vi "Spectral Integration Threshold Ranging.vi"() -> ()   [LabVIEW 2018]
uses:
  <instrlib>/Ocean Optics 2000 4000/Ocean Optics 2000 4000.lvlib
panel:
  out "error out":errorcluster
  in  "Threshold":dbl format="%#_13g"
  out "Peak Wavelength vs Time":cluster{"X":dbl[], "Y":dbl[]}[](graph) caption="XY Graph"
  out "Experiment Length":enum32{"Short", "Long"}(tab)=enum."Long"
  in  "Runtime, s":dbl=20.0
  in  "Maximum Measurement Rate, ms":u32
  in  "Runtime, mins":dbl=20.0
  in  "Maximum Measurement Rate, s":u32=30
  in  "Experiment Length":bool=TRUE
  out "Peak Wavelength Change":cluster{dbl[], dbl[]}(graph)
  out "Integration Change":cluster{dbl[], dbl[]}(graph)
  out "Fitted Target Waveform":cluster{dbl[], dbl[]}(graph)
  out "Target Waveform":cluster{dbl[], dbl[]}(graph)
  in  "?":bool
  out "End Index":i32
  out "Length":i32
  out "Start Index":i32
  out "Calculated Dlambda":dbl[][](array[numeric])
  out "Current Measurement Index":i32
  in  "Wavelength Range":bool
  out "Number of Measurements":dbl
  out "Integration Time":u32
  in  "Intensity Averaging":bool
  out "Integration vs Time":cluster{"Y":dbl[], "Y":dbl[]}[](graph)
  out "Log Data":dbl[][](array[numeric])
  in  "Data Log":bool caption="Log Data"
  in  "File Name":string="Example.xls" caption="add .xls for excel or .tdms, etc"
  in  "Number of Spectrum (Max 5)":i32=5
  in  "Integration Time, ms":dbl=100.0
  in  "Enable Strobe":bool
  out "Spectral Waveform":cluster{dbl[], dbl[]}(graph)
  in  "VISA resource name":refnum<visa-resource-name>
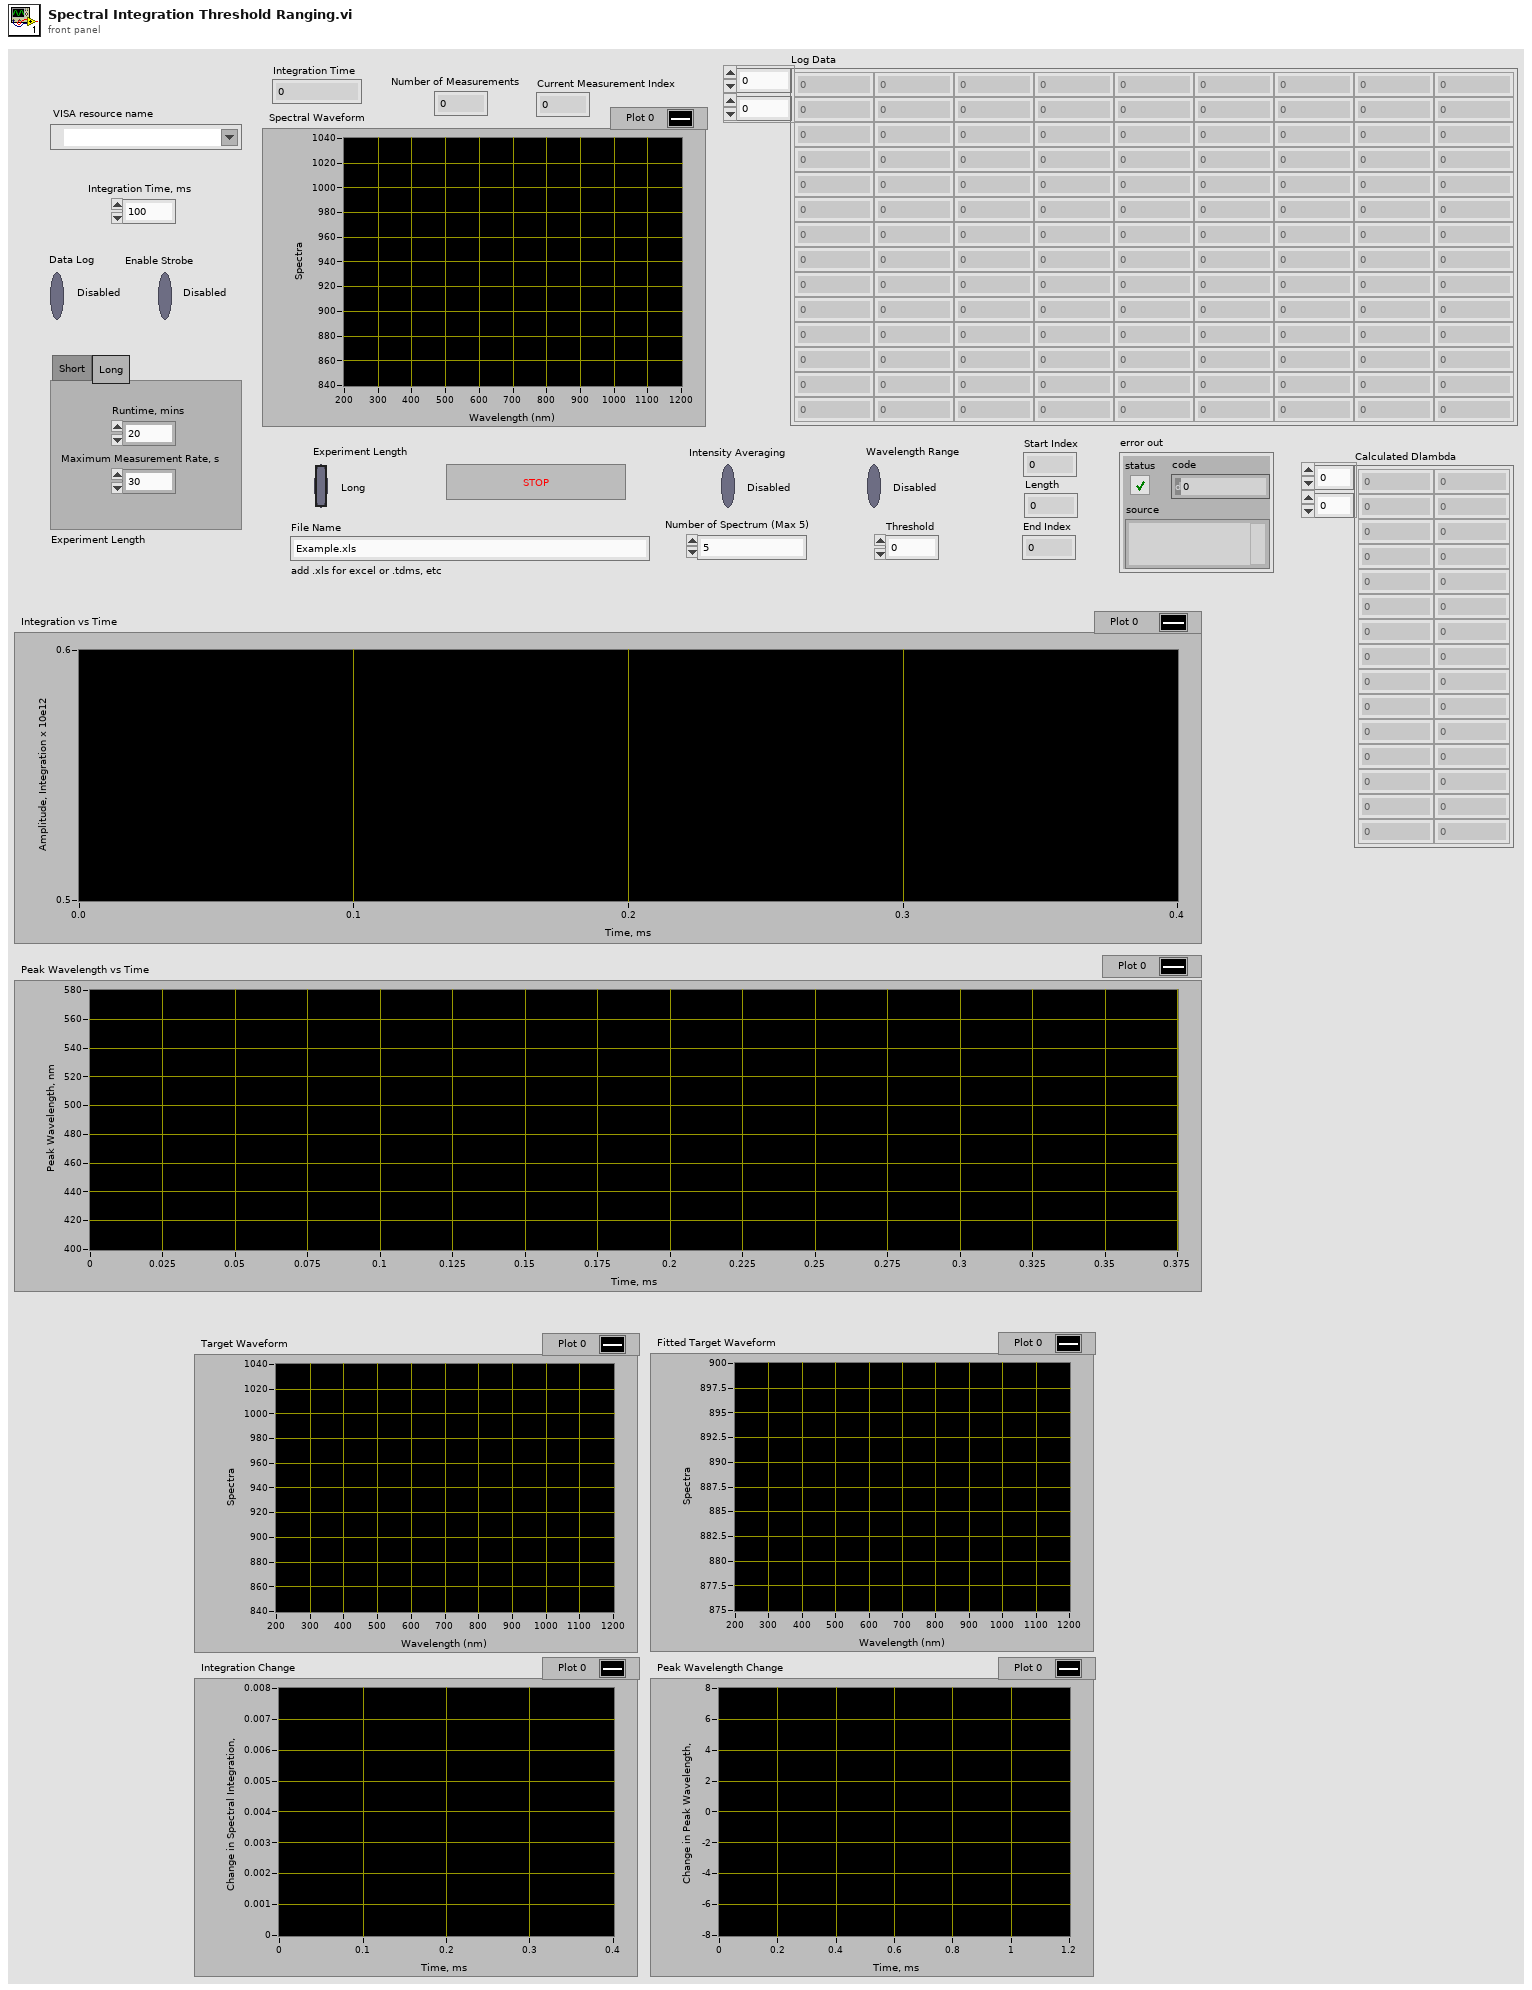
[diagram p1: front panel]
types:
  T1 = cluster{"Wavelength (nm)":dbl[], "Spectrum by Pixel Number":dbl[]}
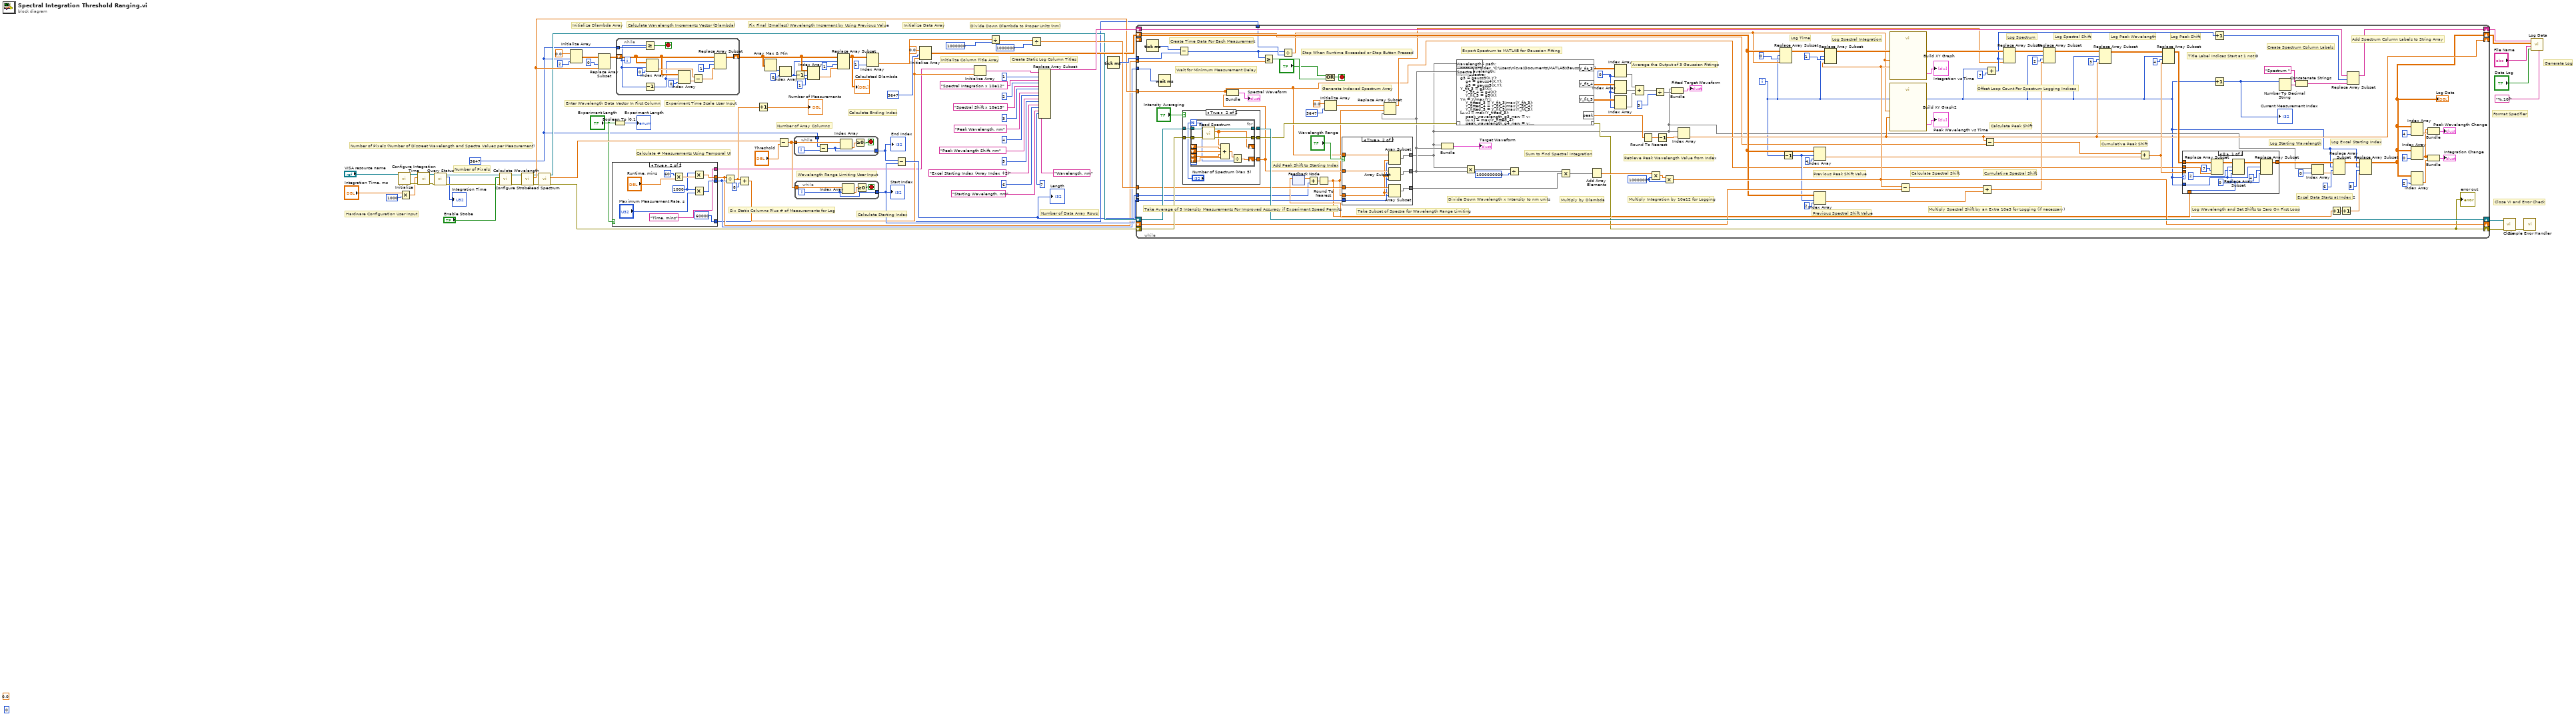
[diagram p0: block diagram]
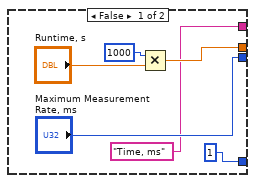
[diagram p2: hidden frame]
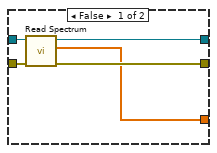
[diagram p5: hidden frame]
diagram:
  w15 = 3647
  (unwired) 0
  (unwired) 0.0 ("element")
  # "Format Specifier"
  # "Number of Pixels"
  # "Calculate Starting Index"
  # "Calculate Ending Index"
  # "Close VI and Error Check"
  # "Six Static Columns Plus # of Measurements for Log"
  # "Number of Array Columns"
  # "Number of Data Array Rows"
  # "Initialize Column Title Array"
  # "Initialize Data Array"
  # "Hardware Configuration User Input"
  # "Generate Log"
  # "Calculate # Measurements Using Temporal UI"
  # "Divide Down Dlambda to Proper Units (nm)"
  # "Number of Pixels (Number of Discreet Wavelength and Spectra Values per Measurement)"
  # "Create Static Log Column Titles"
  # "Experiment Time Scale User Input"
  # "Wavelength Range Limiting User Input"
  # "Fix Final (Smallest) Wavelength Increment by Using Previous Value"
  # "Enter Wavelength Data Vector In First Column"
  # "Initialize Dlambda Array"
  # "Calculate Wavelength Increments Vector (Dlambda)"
  n1 = call <instrlib>:"Initialize.vi"("VISA resource name"="VISA resource name") -> ("error out"=w79:errorcluster, "VISA resource name out"=w80:refnum<visa-resource-name>)  [unwired: 2 in, 7 out]
  n2 = Multiply(x="Integration Time, ms", y=1000) -> (x*y=w78:dbl)
  n3 = call <instrlib>:"Configure Integration Time.vi"("error in (no error)"=w79, "Integration Time (6000)"=w78, "VISA resource name"=w80) -> ("error out"=w77:errorcluster, "VISA resource name out"=w75:refnum<visa-resource-name>)  [unwired: 7 in]
  n4 = call <instrlib>:"Query Status.vi"("VISA resource name"=w75, "error in (no error)"=w77) -> ("VISA resource name out"=w74:refnum<visa-resource-name>, "Integration Time"=→"Integration Time":u32, "error out"=w76:errorcluster)  [unwired: 11 out]
  n5 = call <instrlib>:"Configure Strobe.vi"("error in (no error)"=w76, "Enable Strobe (Disabled)"="Enable Strobe", "VISA resource name"=w74) -> ("error out"=w81:errorcluster, "VISA resource name out"=w82:refnum<visa-resource-name>)  [unwired: 7 out]
  n6 = call <instrlib>:"Calculate Wavelength.vi"("error in (no error)"=w81, "VISA resource name"=w82) -> ("error out"=w28:errorcluster, "Wavelength (nm)"=w31:dbl[], "VISA resource name out"=w30:refnum<visa-resource-name>)  [unwired: 1 in, 6 out]
  n7 = call <instrlib>:"Read Spectrum.vi"("error in (no error)"=w28, "VISA resource name"=w30) -> ("error out"=w27:errorcluster, "Spectrum by Pixel Number"=w26:dbl[], "VISA resource name out"=w29:refnum<visa-resource-name>)  [unwired: 6 in, 1 out]
  n8 = Initialize Array(0.0 ("element"), w15, 2) -> (w58:dbl[][])
  n9 = Replace Array Subset(array=w58, new element=w31, index (col)=0) -> (w56:dbl[][])  [unwired: 1 in]
  n10 = case shown="True" "Experiment Length" {
    tunnel: [w89 w96] -> w16
    tunnel: ["Maximum Measurement Rate, ms" w94] -> w17
    tunnel: [1 60000] -> w9
    tunnel: ["Time, ms" ("string") "Time, mins" ("string")] -> w8
    frame False {
      n11 = Multiply(x=1000, y="Runtime, s") -> (x*y=w89:dbl)
    }
    frame True {
      w93 = 1000
      n12 = Multiply(x=60, y="Runtime, mins") -> (x*y=w97:dbl)
      n13 = Multiply(x=w93, y=w97) -> (x*y=w96:dbl)
      n14 = Multiply(x=w93, y="Maximum Measurement Rate, s") -> (x*y=w94:u32)
    }
  }
  n15 = Boolean To (0,1)(Boolean="Experiment Length") -> (0, 1=→"Experiment Length":i16)
  n16 = while {
    tunnel: w15 -> [w111]
    shift-right: [w105] -> w52
    shift-left: w56 -> [w107]
    i -> [w102]
    stop <- w110 stop-if-true
    n17 = Greater Or Equal?(x=w102, y=w111) -> (x >= y?=w110:bool)
    n18 = Decrement(x=w102) -> (x-1=w103:i32)
    n19 = Index Array(array=w107, index (row)=w102, index (col)=0) -> (element=w109:dbl)
    n20 = Index Array(array=w107, index (row)=w103, index (col)=0) -> (element=w108:dbl)
    n21 = Subtract(x=w109, y=w108) -> (x-y=w104:dbl)
    n22 = Replace Array Subset(array=w107, new element=w104, index (row)=w103, index (col)=1) -> (w105:dbl[][])
  }
  n23 = Divide(x=w16, y=w17) -> (x/y=w33:dbl)
  n24 = Add(x=w33, y=8) -> (x+y=w18:dbl)
  n25 = Increment(x=w33) -> (x+1=→"Number of Measurements":dbl)
  n26 = Array Max & Min(array=w52) -> (min index (indices)=w55:i32[])  [unwired: 3 out]
  n27 = Subtract(x=w26, y="Threshold") -> (x-y=w24:dbl[])
  n28 = Index Array(array=w55, index=0) -> (element=w50:i32)
  n29 = while {
    tunnel: w24 -> [w117]
    tunnel: [w112] -> w23
    tunnel: w15 -> [w114]
    i -> [w113]
    stop <- w115 stop-if-true
    n30 = Subtract(x=w114, y=w113) -> (x-y=w112:i32)
    n31 = Index Array(array=w117, index=w112) -> (element=w116:dbl)
    n32 = Greater Or Equal To 0?(x=w116) -> (x >= 0?=w115:bool)
  }
  "End Index" <- w23
  n33 = Decrement(x=w50) -> (x-1=w54:i32)
  n34 = while {
    tunnel: w24 -> [w121]
    tunnel: [w118] -> w21
    i -> [w118]
    stop <- w119 stop-if-true
    n35 = Index Array(array=w121, index=w118) -> (element=w120:dbl)
    n36 = Greater Or Equal To 0?(x=w120) -> (x >= 0?=w119:bool)
  }
  "Start Index" <- w21
  n37 = Index Array(array=w52, index (row)=w54, index (col)=1) -> (element=w53:dbl)
  n38 = Replace Array Subset(array=w52, new element=w53, index (row)=w50, index (col)=1) -> (w51:dbl[][])
  "Calculated Dlambda" <- w51
  n39 = Index Array(array=w51, index (col)=1) -> (element=w48:dbl[])  [unwired: 1 in]
  n40 = Subtract(x=w23, y=w21) -> (x-y=w20:i32)
  "Length" <- w20
  n41 = Initialize Array(0.0 ("element"), 3647, w18) -> (w40:dbl[][])
  n42 = Initialize Array(w8, w18) -> (w22:string[])
  n43 = Divide(x=w48, y=1000000) -> (x/y=w70:dbl[])
  n44 = Divide(x=w70, y=1000000) -> (x/y=w62:dbl[])
  n45 = Replace Array Subset(array=w22, new element #1="Spectral Integration x 10e12" ("string"), index #1=1, new element #2="Spectral Shift x 10e15" ("string"), index #2=2, new element #3="Peak Wavelength, nm" ("string"), index #3=3, new element #4="Peak Wavelength Shift, nm" ("string"), index #4=4, new element #5="Excel Starting Index (Array Index +2)", index #5=5, new element #6="Starting Wavelength, nm", index #6=6, new element #7="Wavelength, nm", index #7=7) -> (w68:string[])
  n46 = Tick Count (ms)() -> (millisecond timer value=w64:u32)
  n47 = while {
    shift-right: [w228] -> w73
    shift-left: w29 -> [w230]
    shift-right: [w141] -> w72
    shift-left: w27 -> [w229]
    shift-right: [w127] -> w11
    shift-left: w40 -> [w189]
    shift-right: [w180] -> w10
    shift-left: w68 -> [w223]
    tunnel: w64 -> [w218]
    tunnel: w16 -> [w164]
    tunnel: w62 -> [w163]
    tunnel: w31 -> [w135]
    tunnel: w20 -> [w200]
    tunnel: w21 -> [w145]
    shift-right: [w192] -> _
    shift-left: _ -> [w191]
    shift-right: [w151] -> _
    shift-left: _ -> [w149]
    tunnel: w17 -> [w183]
    tunnel: w9 -> [w144]
    i -> [w125]
    stop <- w211 stop-if-true
    w174 = 1000000
    w158 = 0
    # "Log Excel Starting Index"
    # "Excel Data Starts at Index 2"
    # "Log Starting Wavelength"
    # "Generate Indexed Spectrum Array"
    # "Add Peak Shift to Starting Index"
    # "Title Label Indices Start at 1 not 0"
    # "Wait for Minimum Measurement Delay"
    # "Log Wavelength and Set Shifts to Zero On First Loop"
    # "Title Label Indices Start at 1 not 0"
    # "Offset Loop Count For Spectrum Logging Indices"
    # "Log Spectrum"
    # "Log Peak Shift"
    # "Cumulative Peak Shift"
    # "Log Peak Wavelength"
    # "Log Spectral Shift"
    # "Cumulative Spectral Shift"
    # "Multiply Spectral Shift by an Extra 10e3 for Logging (if necessary)"
    # "Log Spectral Integration"
    # "Add Spectrum Column Labels to String Array"
    # "Log Time"
    # "Previous Peak Shift Value"
    # "Previous Spectral Shift Value"
    # "Average the Output of 3 Gaussian Fittings"
    # "Calculate Spectral Shift"
    # "Multiply Integration by 10e12 for Logging"
    # "Sum to Find Spectral Integration"
    # "Calculate Peak Shift"
    # "Retrieve Peak Wavelength Value from Index"
    # "Multiply by Dlambda"
    # "Divide Down Wavelength x Intensity to nm units"
    # "Export Spectrum to MATLAB for Gaussian Fitting"
    # "Stop When Runtime Exceeded or Stop Button Pressed"
    # "Create Time Data For Each Measurement"
    # "Take Average of 5 Intensity Measurements For Improved Accuracy if Experiment Speed Permits"
    # "Take Subset of Spectra for Wavelength Range Limiting"
    # "Create Spectrum Column Labels"
    n48 = Tick Count (ms)() -> (millisecond timer value=w219:u32)
    n49 = Wait (ms)(milliseconds to wait=w183) -> ()  [unwired: 1 out]
    n50 = Subtract(x=w219, y=w218) -> (x-y=w143:u32)
    n51 = case shown="True" "Intensity Averaging" {
      tunnel: w230 -> [w259 w265]
      tunnel: w229 -> [w257 w264]
      tunnel: [w258 w263] -> w228
      tunnel: [w256 w262] -> w208
      tunnel: [w255 w261] -> w159
      frame False {
        n52 = call <instrlib>:"Read Spectrum.vi"("error in (no error)"=w257, "VISA resource name"=w259) -> ("error out"=w256:errorcluster, "Spectrum by Pixel Number"=w255:dbl[], "VISA resource name out"=w258:refnum<visa-resource-name>)  [unwired: 6 in, 1 out]
      }
      frame True {
        n53 = for {
          N: "Number of Spectrum (Max 5)" -> [w266]
          tunnel: w265 -> [w277]
          tunnel: [w275] -> w263
          tunnel: w264 -> [w276]
          tunnel: [w274] -> w262
          shift-right: [w269] -> _
          shift-left: _ -> [w273]
          shift-left: _ -> [w272]
          shift-left: _ -> [w271]
          shift-left: _ -> [w270]
          shift-right: [w268] -> w261
          shift-left: _ -> [_]
          n54 = call <instrlib>:"Read Spectrum.vi"("error in (no error)"=w276, "VISA resource name"=w277) -> ("error out"=w274:errorcluster, "Spectrum by Pixel Number"=w269:dbl[], "VISA resource name out"=w275:refnum<visa-resource-name>)  [unwired: 6 in, 1 out]
          n55 = Compound Arithmetic op=ADD(w269, w273, w272, w271, w270) -> (w267:dbl[])
          n56 = Divide(x=w267, y=w266) -> (x/y=w268:dbl[])
        }
      }
    }
    n57 = Bundle("Wavelength (nm)"=w135, "Spectrum by Pixel Number"=w159) -> (→"Spectral Waveform":T1)  [unwired: 1 out]
    n58 = Greater Or Equal?(x=w143, y=w164) -> (x >= y?=w210:bool)
    n59 = Divide(x=w143, y=w144) -> (x/y=w142:dbl)
    n60 = feedback #1() -> (w146:dbl)  [unwired: 1 in]
    n61 = Add(x=w146, y=w145) -> (x+y=w123:dbl)
    n62 = Round To Nearest(number=w123) -> (nearest integer value=w122:dbl)
    n63 = Or(x="?", y=w210) -> (x .or. y?=w211:bool)
    n64 = Initialize Array(0.0 ("element"), 3647) -> (w138:dbl[])
    n65 = case shown="True" "Wavelength Range" {
      tunnel: w135 -> [w246 w254]
      tunnel: w163 -> [w245 w253]
      tunnel: [w246 w252] -> w126
      tunnel: [w245 w251] -> w162
      tunnel: w200 -> [_ w248]
      tunnel: w122 -> [_ w249]
      tunnel: w159 -> [w244 w250]
      tunnel: [w244 w247] -> w137
      frame False {
      }
      frame True {
        n66 = Array Subset(array=w254, index=w249, length=w248) -> (w252:dbl[])
        n67 = Array Subset(array=w250, index=w249, length=w248) -> (w247:dbl[])
        n68 = Array Subset(array=w253, index=w249, length=w248) -> (w251:dbl[])
      }
    }
    n69 = Replace Array Subset(array=w138, new element=w137, index=w122) -> (w136:dbl[])
    n70 = Bundle("Wavelength (nm)"=w126, "Spectrum by Pixel Number"=w137) -> (→"Target Waveform":T1)  [unwired: 1 out]
    n71 = script code="oldFolder = path;\npath(oldFolder, 'C:\\Users\\nicva\\Documents\\MATLAB\\Gauss Fitting')\nX = Wavelength;\nY = Spectra;\ng3 = gauss3(X,Y);\n    g4 = gauss4(X,Y);\n    g5 = gauss5(X,Y);\nY_fit_3 = g3(X);\n    Y_fit_4 = g4(X);\n    Y_fit_5 = g5(X);\nYn = Y/max(Y);\n    Y_fitted_3 = Y_fit_3/max(Y_fit_3);\n    Y_fitted_4 = Y_fit_4/max(Y_fit_4);\n    Y_fitted_5 = Y_fit_5/max(Y_fit_5);\n[u,v] = max(Y_fitted_3);\n    peak_wavelength_g3_new = v;\n    [u,v] = max(Y_fitted_4);\n    peak_wavelength_g4_new = v;\n    [u,v] = max(Y_fitted_5);\n    peak_wavelength_g5_new = v;\naveraged_wavelengths = [peak_wavelength_g3_new; peak_wavelength_g4_new; peak_wavelength_g5_new];\naveraged_wavelengths = mean(averaged_wavelengths);\npeak = averaged_wavelengths;"("??"=w208, "Spectra"=w137, "Wavelength"=w126) -> ("??"=w141:errorcluster, "peak"=w206:dbl, "Y_fit_3"=w199:dbl[][], "Y_fit_4"=w197:dbl[][], "Y_fit_5"=w196:dbl[][])
    "error out" <- w141
    n72 = Multiply(x=w126, y=w137) -> (x*y=w217:dbl[])
    n73 = Divide(x=w217, y=1000000000) -> (x/y=w216:dbl[])
    n74 = Multiply(x=w216, y=w162) -> (x*y=w212:dbl[])
    n75 = Add Array Elements(numeric array=w212) -> (sum=w214:dbl)
    n76 = Index Array(array=w199, index (col)=w158) -> (element=w198:dbl[])  [unwired: 1 in]
    n77 = Index Array(array=w197, index (col)=w158) -> (element=w195:dbl[])  [unwired: 1 in]
    n78 = Index Array(array=w196, index (col)=w158) -> (element=w194:dbl[])  [unwired: 1 in]
    n79 = Compound Arithmetic op=ADD(w198, w195, w194) -> (w201:dbl[])
    n80 = Round To Nearest(number=w206) -> (nearest integer value=w205:dbl)
    n81 = Multiply(x=w214, y=w174) -> (x*y=w215:dbl)
    n82 = Divide(x=w201, y=3) -> (x/y=w202:dbl[])
    n83 = Decrement(x=w205) -> (x-1=w204:dbl)
    n84 = Multiply(x=w215, y=w174) -> (x*y=w192:dbl)
    n85 = Bundle("Wavelength (nm)"=w126, w202) -> (→"Fitted Target Waveform":cluster{"Wavelength (nm)":dbl[], dbl[]})  [unwired: 1 out]
    n86 = Index Array(array=w126, index=w204) -> (element=w151:dbl)
    n87 = Replace Array Subset(array=w189, new element=w142, index (row)=w125, index (col)=0) -> (w224:dbl[][])
    n88 = Decrement(x=w125) -> (x-1=w154:i32)
    n89 = Index Array(array=w189, index (row)=w154, index (col)=4) -> (element=w155:dbl)
    n90 = Index Array(array=w189, index (row)=w154, index (col)=2) -> (element=w190:dbl)
    n91 = Replace Array Subset(array=w224, new element=w192, index (row)=w125, index (col)=1) -> (w222:dbl[][])
    n92 = call "Build XY Graph"("Y Input"=w192, "X Input"=w142) -> ("XY Graph"=→"Integration vs Time":cluster{"X":dbl[], "Y":dbl[]}[])  [unwired: 8 in, 1 out]
    n93 = call "Build XY Graph2"("Y Input"=w151, "X Input"=w142) -> ("XY Graph"=→"Peak Wavelength vs Time":cluster{"X":dbl[], "Y":dbl[]}[])  [unwired: 8 in, 1 out]
    n94 = Subtract(x=w192, y=w191) -> (x-y=w175:dbl)
    n95 = Add(x=w175, y=w190) -> (x+y=w176:dbl)
    n96 = Subtract(x=w151, y=w149) -> (x-y=w156:dbl)
    n97 = Add(x=w125, y=7) -> (x+y=w152:i32)
    n98 = Replace Array Subset(array=w222, new element=w136, index (col)=w152) -> (w153:dbl[][])  [unwired: 1 in]
    n99 = Replace Array Subset(array=w153, new element=w176, index (row)=w125, index (col)=2) -> (w207:dbl[][])
    n100 = Replace Array Subset(array=w207, new element=w151, index (row)=w125, index (col)=3) -> (w193:dbl[][])
    n101 = Add(x=w156, y=w155) -> (x+y=w147:dbl)
    n102 = Replace Array Subset(array=w193, new element=w147, index (row)=w125, index (col)=4) -> (w181:dbl[][])
    n103 = case shown="0" w125 {
      tunnel: w181 -> [w241 w243]
      tunnel: [w239 w243] -> w128
      tunnel: w125 -> [w238 _]
      tunnel: w135 -> [w236 _]
      tunnel: [w232 w242] -> w148
      tunnel: w147 -> [_ w242]
      frame 0 {
        w232 = 0
        n104 = Replace Array Subset(array=w241, new element=w236, index (col)=7) -> (w237:dbl[][])  [unwired: 1 in]
        n105 = Replace Array Subset(array=w237, new element=w232, index (row)=w238, index (col)=2) -> (w240:dbl[][])
        n106 = Replace Array Subset(array=w240, new element=w232, index (row)=w238, index (col)=4) -> (w239:dbl[][])
      }
      frame 1, Default {
      }
    }
    n107 = feedback-in #1(w148) -> ()
    n108 = Increment(x=w152) -> (x+1=w177:i32)
    n109 = Increment(x=w125) -> (x+1=w179:i32)
    "Current Measurement Index" <- w179
    n110 = Number To Decimal String(number=w179) -> (decimal integer string=w227:string)  [unwired: 1 out]
    n111 = Concatenate Strings("Spectrum " ("string"), w227) -> (w178:string)
    n112 = Index Array(array=w126, index=0) -> (element=w131:dbl)
    n113 = Increment(x=w122) -> (x+1=w130:dbl)
    n114 = Replace Array Subset(array=w128, new element=w131, index (row)=w125, index (col)=6) -> (w134:dbl[][])
    n115 = Increment(x=w130) -> (x+1=w124:dbl)
    n116 = Replace Array Subset(array=w223, new element=w178, index=w177) -> (w180:string[])
    n117 = Replace Array Subset(array=w134, new element=w124, index (row)=w125, index (col)=5) -> (w127:dbl[][])
    "Log Data" <- w127
    n118 = Index Array(array=w127, index (col)=4) -> (element=w185:dbl[])  [unwired: 1 in]
    n119 = Index Array(array=w127, index (col)=0) -> (element=w184:dbl[])  [unwired: 1 in]
    n120 = Index Array(array=w127, index (col)=2) -> (element=w188:dbl[])  [unwired: 1 in]
    n121 = Bundle(w184, w185) -> (→"Peak Wavelength Change":cluster{dbl[], dbl[]})  [unwired: 1 out]
    n122 = Bundle(w184, w188) -> (→"Integration Change":cluster{dbl[], dbl[]})  [unwired: 1 out]
  }
  n123 = call <instrlib>:"Close.vi"("error in (no error)"=w72, "VISA resource name"=w73) -> ("error out"=w71:errorcluster)  [unwired: 9 out]
  n124 = call <vilib>:"Simple Error Handler.vi"("error in (no error)"=w71) -> ()  [unwired: 2 in, 7 out]
  n125 = call "Log Data.vi"("Column Header Array"=w10, "Data Array"=w11, "add .xls for excel or .tdms, etc"="File Name", "Data Log"="Data Log", "Format Specifier (C style)"="%.10f" ("string")) -> ()  [unwired: 5 in]
